vi "BinanceAPI_lastPriceFuture.vi"(0 "BinanceAPI in":refnum<class "BinanceAPI_.lvclass">, 5 "lastPrice":cluster{"symbol (eg. BTCUSDT)":string}, 11 "error in (no error)":errorcluster) -> (4 "BinanceAPI out":refnum<class "BinanceAPI_.lvclass">, 6 "lastPrice":ext, 15 "error out":errorcluster)   [LabVIEW 2022 SP3, in "BinanceAPI_.lvclass"]
doc: "https://binance-docs.github.io/apidocs/futures/en/#symbol-price-ticker"
uses:
  src/BinanceAPI_.lvclass
  src/BinanceAPI_.lvclass/BinanceAPI_.ctl
  <vilib>/regexp/Match Regular Expression.xnode
  <vilib>/httpClient/LabVIEWHTTPClient.lvlib
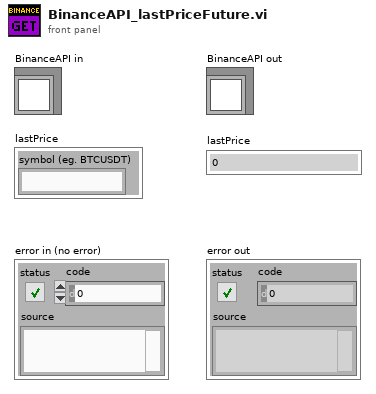
[diagram p1: front panel]
types:
  T1 = typedef "LabVIEWHTTPClient.lvlib/ClientHandle.ctl" = refnum<k1>
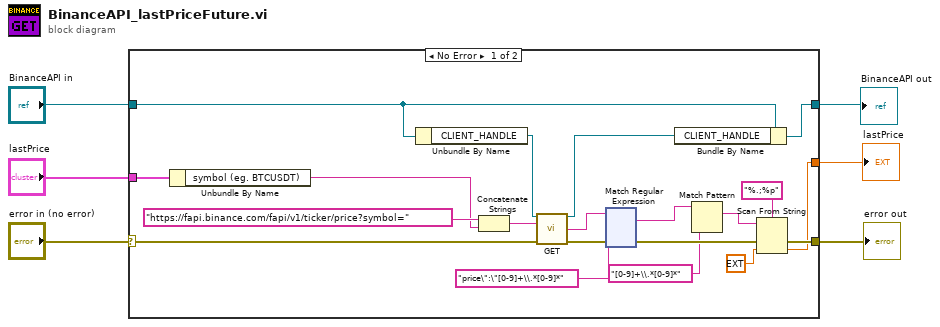
[diagram p0: block diagram]
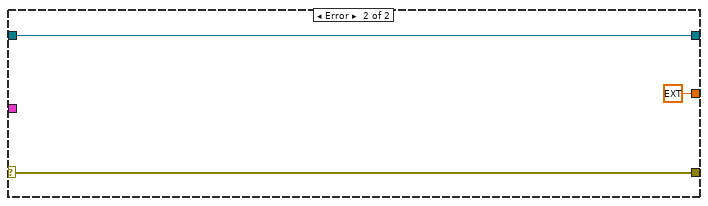
[diagram p2: hidden frame]
diagram:
  n1 = case shown="No Error" "error in (no error)" {
    selector: "error in (no error)" -> [w13 w146]
    tunnel: [w26 w146] -> w6
    tunnel: [w24 ext 0.0 ("default value 1")] -> w5
    tunnel: "BinanceAPI in" -> [w11 w144]
    tunnel: [w10 w144] -> w2
    tunnel: "lastPrice" -> [w8 _]
    frame No Error {
      n2 = Unbundle By Name(w8) -> ("symbol (eg. BTCUSDT)"=w7:string)
      n3 = Unbundle By Name(w11) -> ("CLIENT_HANDLE"=w12:T1)
      n4 = Concatenate Strings("https://fapi.binance.com/fapi/v1/ticker/price?symbol=", w7) -> (w14:string)
      n5 = call <vilib>:"GET.vi"("client handle"=w12, "url"=w14, "error in (no error)"=w13) -> ("client handle out"=w9:T1, "body"=w17:string, "error out"=w18:errorcluster)  [unwired: 9 in, 1 out]
      n6 = xnode "Match Regular Expression"("input string"=w17, "regular expression"="price\":\"[0-9]+\\.*[0-9]*", "error in"=w18) -> ("whole match"=w20:string, "error out"=w25:errorcluster)  [unwired: 3 in, 3 out]
      n7 = Bundle By Name(cluster=w11, "CLIENT_HANDLE"=w9) -> (w10:refnum<class "BinanceAPI_.lvclass">)
      n8 = Match Pattern(string=w20, regular expression="[0-9]+\\.*[0-9]*") -> (match substring=w21:string)  [unwired: 1 in, 3 out]
      n9 = Scan From String(format string="%.;%p", input string=w21, error in=w25, default 1=ext 0.0 ("default value 1")) -> (error out=w26:errorcluster, output 1=w24:ext)  [unwired: 1 in, 2 out]
    }
    frame Error {
    }
  }
  "error out" <- w6
  "lastPrice" <- w5
  "BinanceAPI out" <- w2
